vi "Main.vi"(8 "error in (no error)":errorcluster, 11 "TomoConversionBase in":refnum<class "TomoConversion.lvclass">) -> (0 "error out":errorcluster, 3 "TomoConversionBase out":refnum<class "TomoConversion.lvclass">)   [LabVIEW 2012, in "TomoConversion.lvclass"]
doc: "Main VI of the component."
uses:
  TomoConversion.lvclass
  <vilib>/Distrio/Murmex/Murmex/Murmex.lvclass
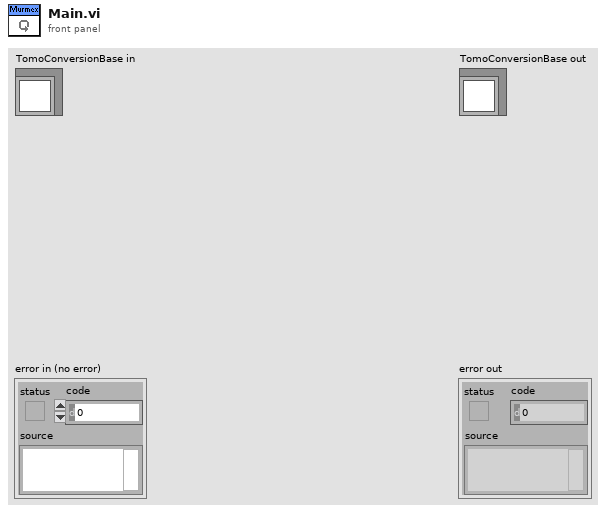
[diagram p1: front panel]
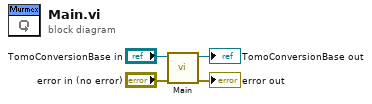
[diagram p0: block diagram]
diagram:
  n1 = call-parent "Main.vi"("error in (no error)"="error in (no error)", "MurmexBase in"="TomoConversionBase in") -> ("error out"=→"error out":errorcluster, "MurmexBase out"=→"TomoConversionBase out":refnum<class "TomoConversion.lvclass">)  [unwired: 8 in]
